vi "NT Write Generic Value.vi"(8 "error in":errorcluster, 9 "Is Control":bool, 10 "Variant":variant, 11 "Name":string="Boolean") -> (0 "error out":errorcluster)   [LabVIEW 2025]
doc: "Write the generic cluster data for a variable into the named entry."
uses:
  <vilib>/Rock Robotics/Network Tables/NT PublishOptions.ctl
  <vilib>/Rock Robotics/Network Tables/NT Datatype.ctl
panel:
  in  "options":T1={"Send All"=FALSE, "Keep Duplicates"=FALSE, "rate (hz)"=10}
  in  "timestamp":u64
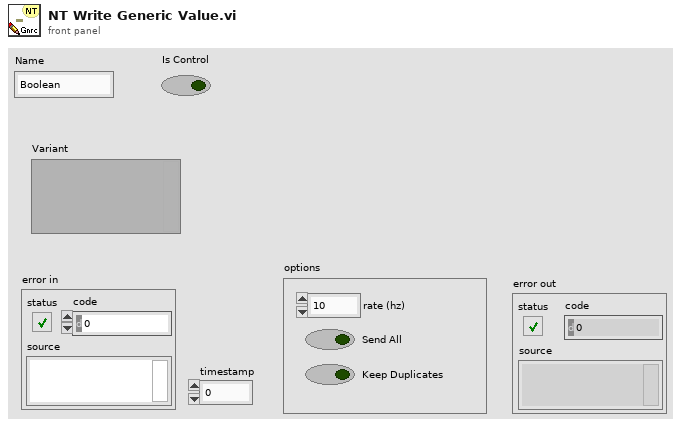
[diagram p1: front panel]
types:
  T1 = typedef "NT PublishOptions.ctl" = cluster{"Send All":bool, "Keep Duplicates":bool, "rate (hz)":u64}
  T2 = typedef "NT Datatype.ctl" = u32
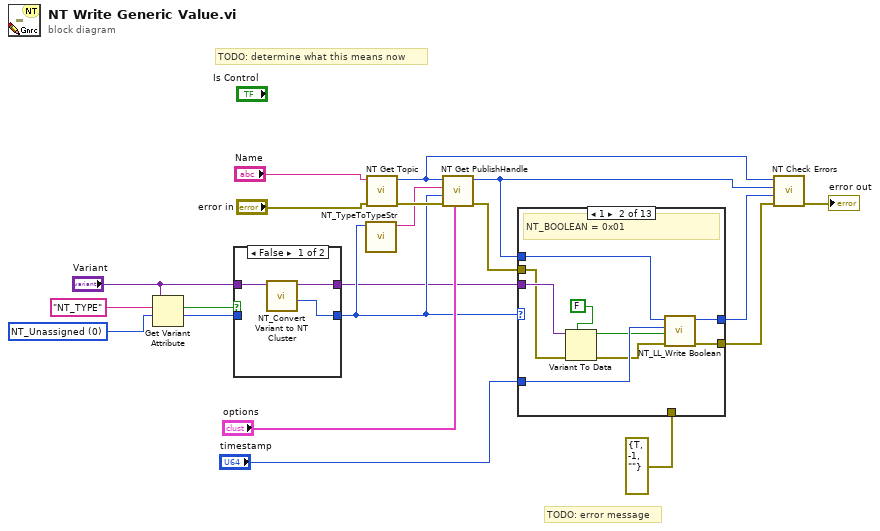
[diagram p0: block diagram]
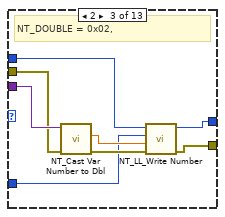
[diagram p4: hidden frame]
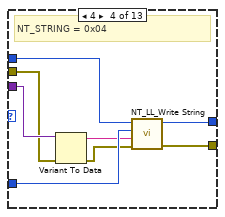
[diagram p5: hidden frame]
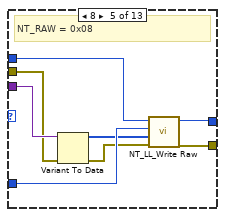
[diagram p6: hidden frame]
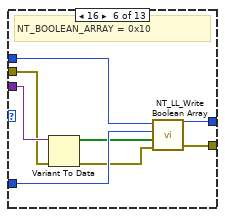
[diagram p7: hidden frame]
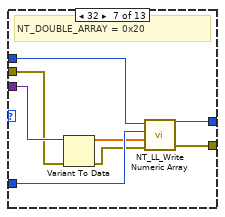
[diagram p8: hidden frame]
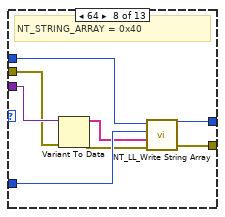
[diagram p9: hidden frame]
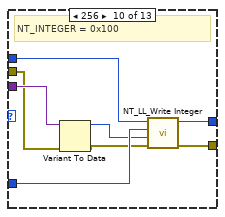
[diagram p11: hidden frame]
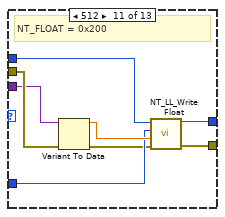
[diagram p12: hidden frame]
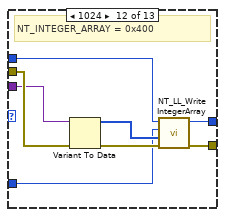
[diagram p13: hidden frame]
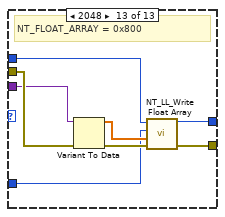
[diagram p14: hidden frame]
diagram:
  w16 = T2 0 items=["NT_Unassigned"=0, "NT_Boolean"=1, "NT_Double"=2, "NT_String"=4, "NT_Raw"=8, "NT_BooleanArray"=16, "NT_DoubleArray"=32, "NT_StringArray"=64, "NT_RPC"=128, "NT_Integer"=256, "NT_Float"=512, "NT_IntegerArray"=1024, "NT_FloatArray"=2048] ("NT_Type")
  # "TODO: error message"
  # "TODO: determine what this means now"
  n1 = Get Variant Attribute(Variant="Variant", name="NT_TYPE", default value (empty Variant)=w16) -> (found=w5:bool, value=w4:T2)  [unwired: 1 in, 2 out]
  n2 = case shown="False" w5 {
    tunnel: w4 -> [_ w25]
    tunnel: [w21 w25] -> w3
    tunnel: "Variant" -> [w23 w24]
    tunnel: [w22 w24] -> w1
    frame False {
      n3 = call <vilib>:"NT_Convert Variant to NT Cluster.vi"("NewVal"=w23) -> ("NT_Type out"=w21:T2, "Value out"=w22:variant)  [unwired: 9 in]
    }
    frame True {
    }
  }
  n4 = call <vilib>:"NT_TypeToTypeStr.vi"("type"=w3) -> ("typeStr"=w6:string)  [unwired: 10 in]
  n5 = call <vilib>:"NT Get Topic.vi"("error in (no error)"="error in", "name"="Name") -> ("error out"=w20:errorcluster, "topicHandle"=w8:u32)  [unwired: 8 in]
  n6 = call <vilib>:"NT Get PublishHandle.vi"("options"="options", "error in (no error)"=w20, "NT_Type"=w3, "description"=w6, "topicHandle"=w8) -> ("error out"=w12:errorcluster, "publishHandle"=w7:u32)  [unwired: 5 in]
  n7 = case shown="1" w3 {
    tunnel: "timestamp" -> [_ w32 w38 w48 w56 w64 w72 w80 _ w89 w94 w102 w110]
    tunnel: w1 -> [_ w31 w43 w47 w55 w63 w71 w79 _ w92 w96 w105 w112]
    tunnel: w12 -> [_ w30 w42 w45 w53 w61 w68 w76 _ w91 w97 w106 w113]
    tunnel: [w26 w35 w40 w50 w58 w66 w75 w82 w84 w85 w100 w107 w115] -> w9
    tunnel: [_ w34 w36 w51 w59 w67 w74 w83 _ w86 w99 w108 w116] -> w11
    tunnel: w7 -> [_ w33 w37 w49 w57 w65 w73 w81 _ w90 w98 w101 w109]
    tunnel: errorcluster {"status"=TRUE, "code"=-1, "source"=""} ("error out") -> [w26 _ _ _ _ _ _ _ w84 _ _ _ _]
    frame 0, Default {
      # "NT_UNASSIGNED=0"
    }
    frame 1 {
      # "NT_BOOLEAN = 0x01"
      n8 = Variant To Data(error in=w30, type=FALSE ("Owning Write"), Variant=w31) -> (data=w28:bool, error out=w29:errorcluster)
      n9 = call <vilib>:"NT_LL_Write Boolean.vi"("error in (no error)"=w29, "Boolean"=w28, "timestamp"=w32, "publishHandle"=w33) -> ("error out"=w35:errorcluster, "success"=w34:u32)  [unwired: 6 in]
    }
    frame 2 {
      # "NT_DOUBLE = 0x02,"
      n10 = call <vilib>:"NT_Cast Var Number to Dbl.vi"("error in (no error)"=w42, "NewVal"=w43) -> ("error out"=w41:errorcluster, "Numeric"=w39:dbl)  [unwired: 8 in]
      n11 = call <vilib>:"NT_LL_Write Number.vi"("error in (no error)"=w41, "value"=w39, "timestamp"=w38, "publishHandle"=w37) -> ("error out"=w40:errorcluster, "success"=w36:u32)  [unwired: 6 in]
    }
    frame 4 {
      # "NT_STRING = 0x04"
      n12 = Variant To Data(error in=w45, Variant=w47) -> (data=w46:string, error out=w44:errorcluster)  [unwired: 1 in]
      n13 = call <vilib>:"NT_LL_Write String.vi"("error in (no error)"=w44, "value"=w46, "timestamp"=w48, "publishHandle"=w49) -> ("error out"=w50:errorcluster, "success"=w51:u32)  [unwired: 6 in]
    }
    frame 8 {
      # "NT_RAW = 0x08"
      n14 = Variant To Data(error in=w53, Variant=w55) -> (data=w54:u8[], error out=w52:errorcluster)  [unwired: 1 in]
      n15 = call <vilib>:"NT_LL_Write Raw.vi"("error in (no error)"=w52, "unsigned byte array"=w54, "timestamp"=w56, "publishHandle"=w57) -> ("error out"=w58:errorcluster, "success"=w59:u32)  [unwired: 6 in]
    }
    frame 16 {
      # "NT_BOOLEAN_ARRAY = 0x10"
      n16 = Variant To Data(error in=w61, Variant=w63) -> (data=w62:bool[], error out=w60:errorcluster)  [unwired: 1 in]
      n17 = call <vilib>:"NT_LL_Write Boolean Array.vi"("error in (no error)"=w60, "value"=w62, "timestamp"=w64, "publishHandle"=w65) -> ("error out"=w66:errorcluster, "success"=w67:u32)  [unwired: 6 in]
    }
    frame 32 {
      # "NT_DOUBLE_ARRAY = 0x20"
      n18 = Variant To Data(error in=w68, Variant=w71) -> (data=w70:dbl[], error out=w69:errorcluster)  [unwired: 1 in]
      n19 = call <vilib>:"NT_LL_Write Numeric Array.vi"("error in (no error)"=w69, "value"=w70, "timestamp"=w72, "publishHandle"=w73) -> ("error out"=w75:errorcluster, "success"=w74:u32)  [unwired: 6 in]
    }
    frame 64 {
      # "NT_STRING_ARRAY = 0x40"
      n20 = Variant To Data(error in=w76, Variant=w79) -> (data=w78:string[], error out=w77:errorcluster)  [unwired: 1 in]
      n21 = call <vilib>:"NT_LL_Write String Array.vi"("error in (no error)"=w77, "value"=w78, "timestamp"=w80, "publishHandle"=w81) -> ("error out"=w82:errorcluster, "success"=w83:u32)  [unwired: 6 in]
    }
    frame 128 {
      # "NT_RPC = 0x80"
    }
    frame 256 {
      # "NT_INTEGER = 0x100"
      n22 = Variant To Data(error in=w91, Variant=w92) -> (data=w88:i64, error out=w87:errorcluster)  [unwired: 1 in]
      n23 = call <vilib>:"NT_LL_Write Integer.vi"("error in (no error)"=w87, "value"=w88, "timestamp"=w89, "publishHandle"=w90) -> ("error out"=w85:errorcluster, "success"=w86:u32)  [unwired: 6 in]
    }
    frame 512 {
      # "NT_FLOAT = 0x200"
      n24 = Variant To Data(error in=w97, Variant=w96) -> (data=w95:sgl, error out=w93:errorcluster)  [unwired: 1 in]
      n25 = call <vilib>:"NT_LL_Write Float.vi"("error in (no error)"=w93, "value"=w95, "timestamp"=w94, "publishHandle"=w98) -> ("error out"=w100:errorcluster, "success"=w99:u32)  [unwired: 6 in]
    }
    frame 1024 {
      # "NT_INTEGER_ARRAY = 0x400"
      n26 = Variant To Data(error in=w106, Variant=w105) -> (data=w103:i64[], error out=w104:errorcluster)  [unwired: 1 in]
      n27 = call <vilib>:"NT_LL_Write IntegerArray.vi"("error in (no error)"=w104, "value"=w103, "timestamp"=w102, "publishHandle"=w101) -> ("error out"=w107:errorcluster, "success"=w108:u32)  [unwired: 6 in]
    }
    frame 2048 {
      # "NT_FLOAT_ARRAY = 0x800"
      n28 = Variant To Data(error in=w113, Variant=w112) -> (data=w111:sgl[], error out=w114:errorcluster)  [unwired: 1 in]
      n29 = call <vilib>:"NT_LL_Write Float Array.vi"("error in (no error)"=w114, "value"=w111, "timestamp"=w110, "publishHandle"=w109) -> ("error out"=w115:errorcluster, "success"=w116:u32)  [unwired: 6 in]
    }
  }
  n30 = call <vilib>:"NT Check Errors.vi"("error in (no error)"=w9, "success"=w11, "pubSubHandle"=w7, "topicHandle"=w8) -> ("error out"=→"error out":errorcluster)  [unwired: 7 in]
